vi "Error Converter (ErrCode or Status).vi"(8 "error in (no error)":errorcluster, 10 "handle in":u64, 11 "error code":i32) -> (0 "error out":errorcluster)   [LabVIEW 2020, in "Ballard ARINC 429 Hardware API.lvlib"]
uses:
  <instrlib>/BTICardLib/Public/Controls/Error Info.ctl
  Ballard ARINC 429 Hardware API.lvlib
  <instrlib>/BTICardLib/BTICardLV.lvlib
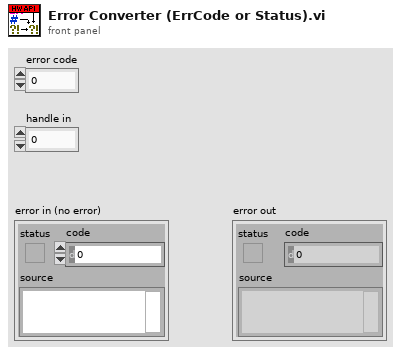
[diagram p1: front panel]
types:
  T1 = typedef "BTICardLV.lvlib/Error Info.ctl" = u32
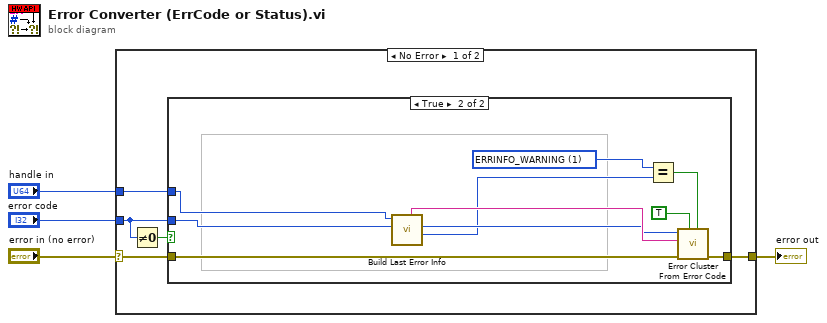
[diagram p0: block diagram]
diagram:
  n1 = case shown="No Error" "error in (no error)" {
    selector: "error in (no error)" -> [w9 w21]
    tunnel: [w8 w21] -> w3
    tunnel: "error code" -> [w6 _]
    tunnel: "handle in" -> [w7 _]
    frame No Error {
      n2 = Not Equal To 0?(x=w6) -> (x != 0?=w5:bool)
      n3 = case shown="True" w5 {
        tunnel: w9 -> [w10 w20]
        tunnel: w6 -> [_ w16]
        tunnel: [w10 w19] -> w8
        tunnel: w7 -> [_ w14]
        frame False {
        }
        frame True {
          w12 = T1 1 items=["ERRINFO_ERROR", "ERRINFO_WARNING", "ERRINFO_INFO"] ("error info")
          n4 = call "Build Last Error Info.vi"("error code in"=w16, "handle in"=w14) -> ("error info"=w13:T1, "error code out"=w15:i32, "error string out"=w17:string)  [unwired: 5 in, 2 out]
          n5 = Equal?(x=w12, y=w13) -> (x = y?=w11:bool)
          n6 = call <vilib>:"Error Cluster From Error Code.vi"("is warning? (False)"=w11, "show call chain? (False)"=TRUE, "error in (no error)"=w20, "error message (\"\")"=w17, "error code (0)"=w15) -> ("error out"=w19:errorcluster)  [unwired: 4 in]
        }
      }
    }
    frame Error {
    }
  }
  "error out" <- w3
